vi "Compile.vi"(4 "LocalCompiledDir":path, 5 "Message Box":refnum<vi>, 6 "Compilation Type":T1, 7 "DevMode":bool, 8 "error in":errorcluster, 11 "VI Path":path) -> (0 "error out":errorcluster, 3 "Source Dir":path)   [LabVIEW 2014]
uses:
  Custom Controls/CompileType.ctl
  Compiler/RasPi Compiler.lvclass/RasPi Compiler.ctl
  Compiler/RasPi Compiler.lvclass
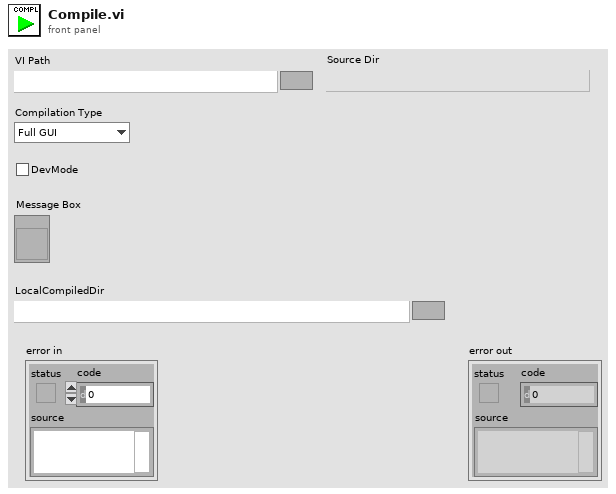
[diagram p1: front panel]
types:
  T1 = typedef "CompileType.ctl" = enum16{"Full GUI", "Console App"}
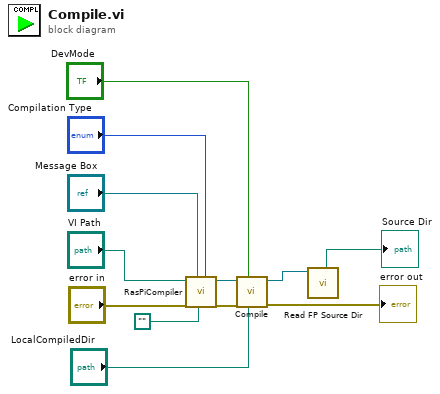
[diagram p0: block diagram]
diagram:
  n1 = call "RasPiCompiler.vi"("Compilation Type"="Compilation Type", "Build Path"=path "", "Message Box"="Message Box", "error in"="error in", "VI Path"="VI Path") -> ("error out"=w11:errorcluster, "RasPi Compiler out"=w3:refnum<class "RasPi Compiler.lvclass">)  [unwired: 5 in]
  n2 = call "Compile.vi"("LocalCompiledDir"="LocalCompiledDir", "DevMode"="DevMode", "error in"=w11, "RasPi Compiler in"=w3) -> ("error out"=→"error out":errorcluster, "RasPi Compiler out"=w10:refnum<class "RasPi Compiler.lvclass">)  [unwired: 6 in]
  n3 = call "Read FP Source Dir.vi"("RasPi Compiler in"=w10) -> ("FP Source Dir"=→"Source Dir":path)  [unwired: 7 in, 1 out]
